vi "PFE Driver.vi"(5 "PFE Configuration (\"\")":string, 6 "Drv Refnum":T1, 7 "PFE Command":T2, 8 "error in (no error)":errorcluster, 10 "PFE Position In":variant) -> (0 "error out":errorcluster, 1 "PFE Flat Output":string, 2 "PFE Position Out":variant, 4 "dup Drv Refnum":T1)   [LabVIEW 2011]
uses:
  PFE Command.ctl
  PFE Driver Ref.ctl
panel:
  in  "DEBUG?":bool
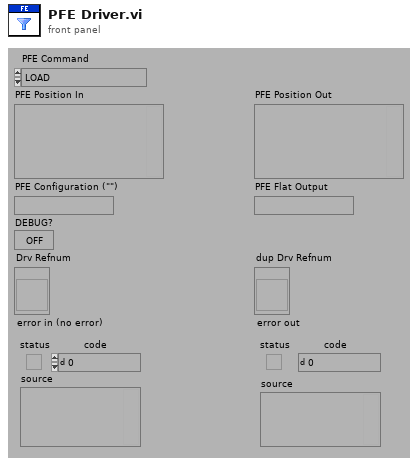
[diagram p1: front panel]
types:
  T1 = typedef "PFE Driver Ref.ctl" = refnum<vi>
  T2 = typedef "PFE Command.ctl" = enum16{"LOAD", "INITIALIZE", "PRESET", "SET STIMULUS", "GET STIMULUS", "GET INFO", "RELEASE", "UNLOAD"}
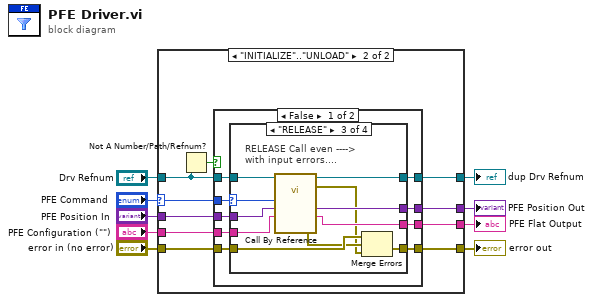
[diagram p0: block diagram]
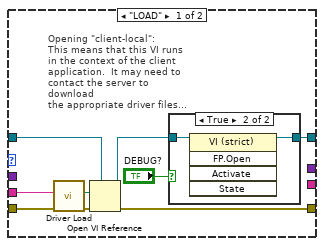
[diagram p2: hidden frame]
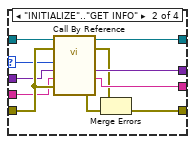
[diagram p5: hidden frame]
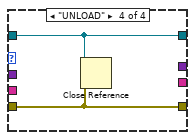
[diagram p6: hidden frame]
diagram:
  n1 = case shown="\"INITIALIZE\"..\"UNLOAD\"" "PFE Command" {
    selector: "PFE Command" -> [_ w24]
    tunnel: "error in (no error)" -> [w18 w31]
    tunnel: "PFE Position In" -> [_ w30]
    tunnel: [_ w29] -> w7
    tunnel: [w17 w28] -> w6
    tunnel: "PFE Configuration (\"\")" -> [w16 w27]
    tunnel: [_ w26] -> w4
    tunnel: [w15 w25] -> w3
    tunnel: "Drv Refnum" -> [w14 w23]
    frame "LOAD" {
      # "Opening \"client-local\":\nThis means that this VI runs\nin the context of the client\napplication.  It may need to\ncontact the server to download\nthe appropriate driver files..."
      n2 = call "Driver Load.vi"("error in (no error)"=w18, "DriverID DriverType (\"\")"=w16) -> ("error out"=w10:errorcluster, "Driver Component Path"=w11:path)  [unwired: 1 in, 7 out]
      n3 = Open VI Reference(type specifier VI Refnum (for type only)=w14, vi path=w11, error in (no error)=w10) -> (vi reference=w13:T1, error out=w17:errorcluster)  [unwired: 3 out]
      n4 = case shown="True" "DEBUG?" {
        tunnel: w13 -> [w19 w21]
        tunnel: [w19 w20] -> w15
        frame False {
        }
        frame True {
          n5 = invoke class="VI (strict)" method="FP.Open"(reference=w21) -> (reference out=w20:T1)  [unwired: 4 in, 4 out]
        }
      }
    }
    frame "INITIALIZE".."UNLOAD" {
      n6 = Not A Number/Path/Refnum?(number/path/refnum=w23) -> (NaN/Path/Refnum?=w22:bool)
      n7 = case shown="False" w22 {
        tunnel: w31 -> [w40 w67]
        tunnel: w30 -> [w39 _]
        tunnel: [w38 _] -> w29
        tunnel: [w37 w67] -> w28
        tunnel: w27 -> [w36 _]
        tunnel: [w35 _] -> w26
        tunnel: [w34 w68] -> w25
        tunnel: w23 -> [w33 w68]
        tunnel: w24 -> [w32 _]
        frame False {
          n8 = case shown="\"RELEASE\"" w32 {
            selector: w32 -> [_ w43 w55 _]
            tunnel: w40 -> [w42 w51 w59 w65]
            tunnel: w39 -> [_ w48 w61 _]
            tunnel: [_ w50 w63 _] -> w38
            tunnel: [w42 w53 w64 w65] -> w37
            tunnel: w36 -> [_ w47 w60 _]
            tunnel: [_ w49 w62 _] -> w35
            tunnel: [w41 w52 w54 w66] -> w34
            tunnel: w33 -> [w41 w44 w56 w66]
            frame "LOAD", Default {
              # "This will not ever run."
            }
            frame "INITIALIZE".."GET INFO" {
              n9 = call-by-ref "?"(reference=w44, error in=w51, "error in (no error)"=w51, "SWI Configuration (\"\")"=w47, "SWI Position In"=w48, "SWI Command"=w43) -> (reference out=w52:T1, error out=w45:errorcluster, 0:"error out"=w46:errorcluster, "SWI Flat Output"=w49:string, "SWI Position Out"=w50:variant)  [unwired: 5 in]
              n10 = Merge Errors(w45, w46) -> (w53:errorcluster)
            }
            frame "RELEASE" {
              # "RELEASE Call even ---->\nwith input errors...."
              n11 = call-by-ref "?"(reference=w56, "SWI Configuration (\"\")"=w60, "SWI Position In"=w61, "SWI Command"=w55) -> (reference out=w54:T1, error out=w57:errorcluster, 0:"error out"=w58:errorcluster, "SWI Flat Output"=w62:string, "SWI Position Out"=w63:variant)  [unwired: 7 in]
              n12 = Merge Errors(w59, w58, w57) -> (w64:errorcluster)
            }
            frame "UNLOAD" {
              n13 = Close Reference(reference=w66, error in (no error)=w65) -> ()  [unwired: 1 out]
            }
          }
        }
        frame True {
          # "If the reference is not valid\nno operation is performed."
        }
      }
    }
  }
  "error out" <- w6
  "PFE Position Out" <- w7
  "PFE Flat Output" <- w4
  "dup Drv Refnum" <- w3
